vi "Wait ms.vi"(5 "Wait on error? (F)":bool, 7 "Wait (1000 ms)":u32=1000, 8 "error in (no error)":errorcluster, 11 "VISA Session":refnum<visa-resource-name>) -> (0 "error out":errorcluster, 3 "VISA Session out":refnum<visa-resource-name>)   [LabVIEW 2017]
doc: "Anritsu LabVIEW Toolkit\n\nPauses execution for the given number of milliseconds.\n\nINPUTS\n Wait - number of milliseconds to pause.\n Wait on error? - whether or not execution will still pause if an error is passed in."
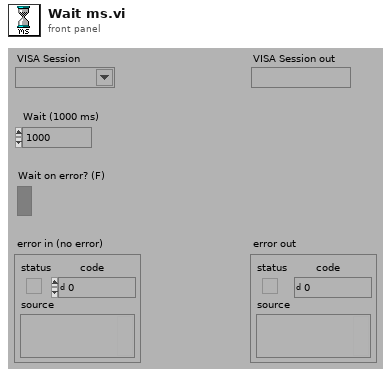
[diagram p1: front panel]
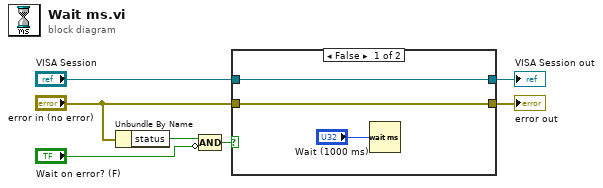
[diagram p0: block diagram]
diagram:
  n1 = Unbundle By Name("error in (no error)") -> ("status"=w3:bool)
  n2 = Compound Arithmetic op=AND(w3, invert "Wait on error? (F)") -> (w1:bool)
  n3 = case shown="False" w1 {
    tunnel: "VISA Session" -> [w9 w12]
    tunnel: [w9 w12] -> w6
    tunnel: [w8 w11] -> w5
    tunnel: "error in (no error)" -> [w8 w11]
    frame False {
      n4 = Wait (ms)(milliseconds to wait="Wait (1000 ms)") -> ()  [unwired: 1 out]
    }
    frame True {
    }
  }
  "VISA Session out" <- w6
  "error out" <- w5
